vi "Get AI Status.vi"(0 "Module Ref":refnum<class "Modbus Master.lvclass">, 11 "error in (no error)":errorcluster) -> (4 "Modbus master out":refnum<class "Modbus Master.lvclass">, 15 "error out":errorcluster)   [LabVIEW 2024]
doc: "Read back analogue input status registers."
uses:
  <vilib>/NI/Modbus Library/API/Master/Modbus Master.lvclass
  Support VIs/AI Status Cluster.ctl
panel:
  out "AI Status":T1[](array[typedef])
  # "Channel 0"
  # "Channel 1"
  # "Channel 2"
  # "Channel 3"
  # "Channel 4"
  # "Channel 5"
  # "Channel 6"
  # "Channel 7"
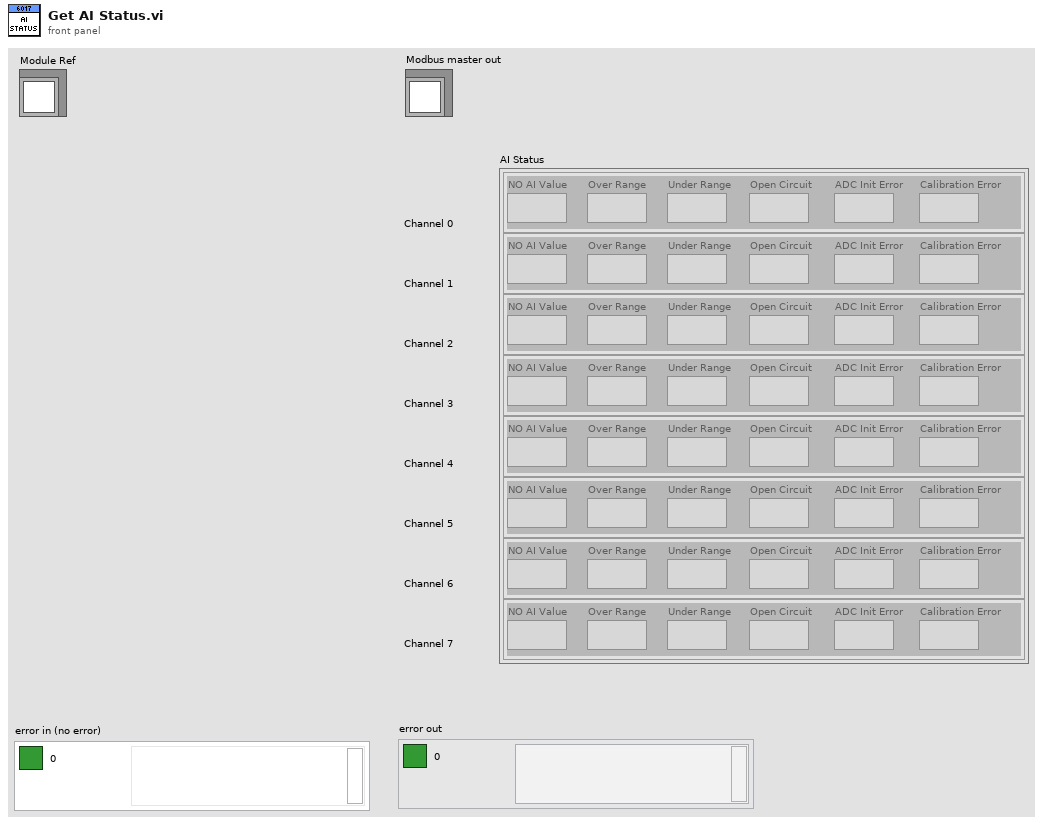
[diagram p1: front panel]
types:
  T1 = typedef "AI Status Cluster.ctl" = cluster{"NO AI Value":bool, "Over Range":bool, "Under Range":bool, "Open Circuit":bool, "ADC Init Error":bool, "Calibration Error":bool}
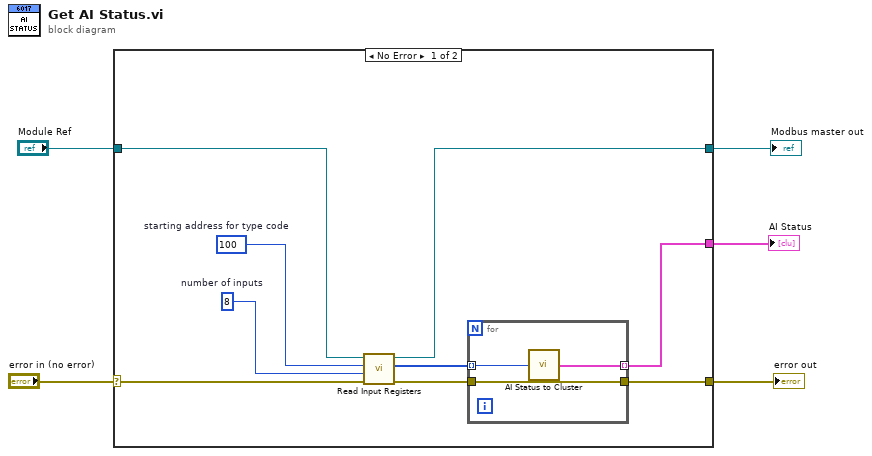
[diagram p0: block diagram]
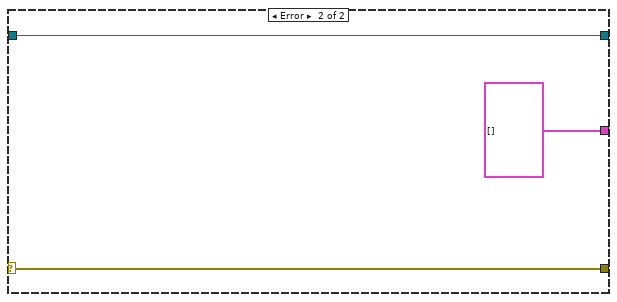
[diagram p2: hidden frame]
diagram:
  n1 = case shown="No Error" "error in (no error)" {
    selector: "error in (no error)" -> [w14 w19]
    tunnel: "Module Ref" -> [w12 w20]
    tunnel: [w7 w19] -> w3
    tunnel: [w13 w20] -> w2
    tunnel: [w6 T1[] []] -> w1
    frame No Error {
      w10 = u16 8  # number of inputs
      w11 = u16 100  # starting address for type code
      n2 = call-dynamic "Read Input Registers.vi"("error in"=w14, "number of inputs"=w10, "starting address"=w11, "Modbus master in"=w12) -> ("error out"=w8:errorcluster, "register values"=w9:u16[], "Modbus master out"=w13:refnum<class "Modbus Master.lvclass">)  [unwired: 5 in]
      n3 = for {
        tunnel: w9 -> [w16] mode=indexing
        tunnel: w8 -> [w17]
        tunnel: [w17] -> w7
        tunnel: [w15] -> w6 mode=indexing
        n4 = call "AI Status to Cluster.vi"("AI Status Register"=w16) -> ("AI Status Cluster"=w15:T1)
      }
    }
    frame Error {
    }
  }
  "error out" <- w3
  "Modbus master out" <- w2
  "AI Status" <- w1
